vi "Average Array at Interval (SubVI).vi"(0 "Signals IN":dbl[](array[numeric]), 7 "Enable":bool=TRUE, 12 "Sample Interval [sec]":dbl, 13 "Reset Averages":bool) -> (4 "Signals OUT":dbl[](array[numeric]), 8 "Ave Size":i32)   [LabVIEW 2012]
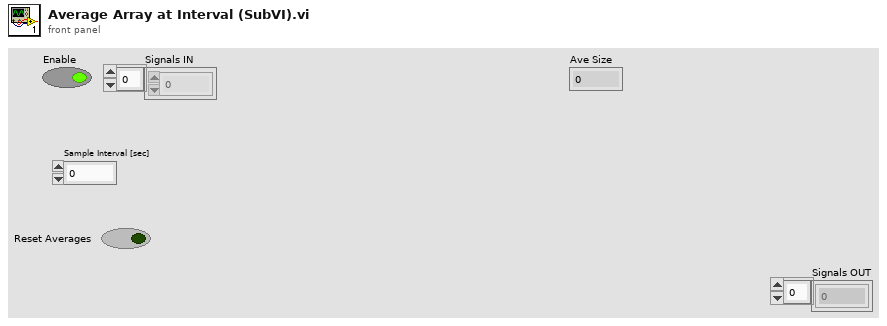
[diagram p1: front panel]
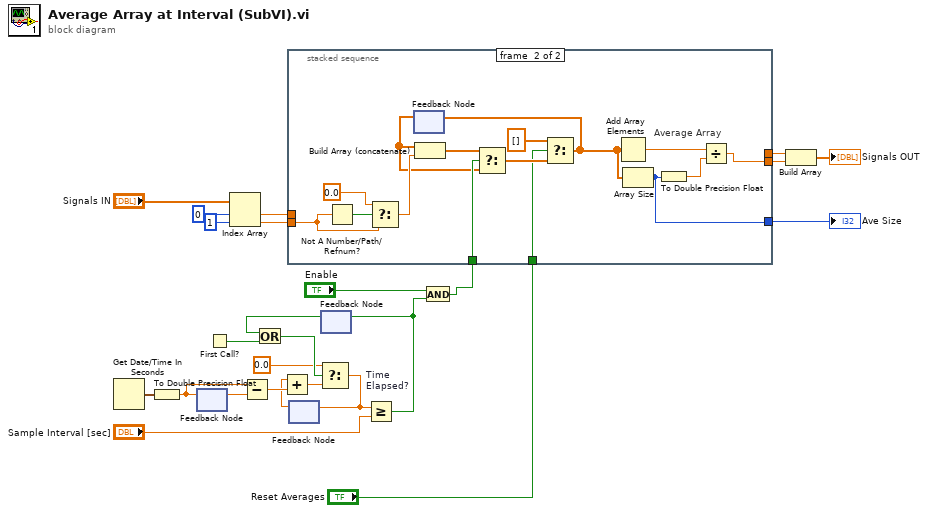
[diagram p0: block diagram]
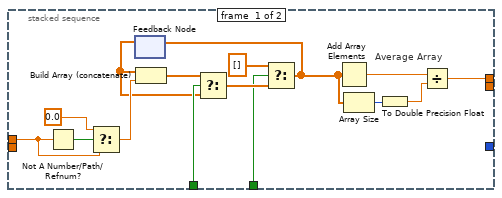
[diagram p2: hidden frame]
diagram:
  n1 = Get Date/Time In Seconds() -> (seconds since 1Jan1904=w17:timestamp)
  n2 = To Double Precision Float(number=w17) -> (double precision float=w18:dbl)
  n3 = feedback #1() -> (w16:dbl)  [unwired: 1 in]
  n4 = feedback-in #1(w18) -> ()
  n5 = First Call?() -> (First Call?: T/F=w24:bool)
  n6 = Index Array(array="Signals IN", index #1=0, index #2=1) -> (element #1=w9:dbl, element #2=w8:dbl)
  n7 = Subtract(x=w18, y=w16) -> (x-y=w19:dbl)
  n8 = feedback #2() -> (w15:dbl)  [unwired: 1 in]
  n9 = Add(x=w15, y=w19) -> (x+y=w20:dbl)
  n10 = feedback #3() -> (w25:bool)  [unwired: 1 in]
  n11 = Or(x=w25, y=w24) -> (x .or. y?=w23:bool)
  n12 = Select(t=0.0, s=w23, f=w20) -> (s? t:f=w22:dbl)
  n13 = feedback-in #2(w22) -> ()
  n14 = Greater Or Equal? "Time\nElapsed?"(x=w22, y="Sample Interval [sec]") -> (x >= y?=w3:bool)
  n15 = feedback-in #3(w3) -> ()
  n16 = And(x="Enable", y=w3) -> (x .and. y?=w2:bool)
  n17 = stacked-sequence {
    tunnel: w2 -> [w36 w52]
    tunnel: [w30 _] -> w13
    tunnel: "Reset Averages" -> [w27 w44]
    tunnel: [_ w43] -> w12
    tunnel: w9 -> [w26 _]
    tunnel: w8 -> [_ w42]
    tunnel: [_ w41] -> w5
    frame #0 {
      # "Average Array"
      n18 = Not A Number/Path/Refnum?(number/path/refnum=w26) -> (NaN/Path/Refnum?=w33:bool)
      n19 = Select(t=0.0, s=w33, f=w26) -> (s? t:f=w31:dbl)
      n20 = feedback #4() -> (w28:dbl[])  [unwired: 1 in]
      n21 = Build Array (concatenate)(w28, w31) -> (w37:dbl[])
      n22 = Select(t=w37, s=w36, f=w28) -> (s? t:f=w34:dbl[])
      n23 = Select(t=dbl[] [], s=w27, f=w34) -> (s? t:f=w29:dbl[])
      n24 = feedback-in #4(w29) -> ()
      n25 = Add Array Elements(numeric array=w29) -> (sum=w39:dbl)
      n26 = Array Size(array=w29) -> (size(s)=w38:i32)
      n27 = To Double Precision Float(number=w38) -> (double precision float=w40:dbl)
      n28 = Divide(x=w39, y=w40) -> (x/y=w30:dbl)
    }
    frame #1 {
      # "Average Array"
      n29 = Not A Number/Path/Refnum?(number/path/refnum=w42) -> (NaN/Path/Refnum?=w49:bool)
      n30 = Select(t=0.0, s=w49, f=w42) -> (s? t:f=w47:dbl)
      n31 = feedback #5() -> (w45:dbl[])  [unwired: 1 in]
      n32 = Build Array (concatenate)(w45, w47) -> (w53:dbl[])
      n33 = Select(t=w53, s=w52, f=w45) -> (s? t:f=w50:dbl[])
      n34 = Select(t=dbl[] [], s=w44, f=w50) -> (s? t:f=w46:dbl[])
      n35 = feedback-in #5(w46) -> ()
      n36 = Add Array Elements(numeric array=w46) -> (sum=w54:dbl)
      n37 = Array Size(array=w46) -> (size(s)=w41:i32)
      n38 = To Double Precision Float(number=w41) -> (double precision float=w55:dbl)
      n39 = Divide(x=w54, y=w55) -> (x/y=w43:dbl)
    }
  }
  "Ave Size" <- w5
  n40 = Build Array(w13, w12) -> (→"Signals OUT":dbl[])
